vi "Test YOLO.vi"() -> ()   [LabVIEW 2017]
doc: "Created IvanLis by LabVIEW Portal\nProfile: http://labviewportal.org/memberlist.php?mode=viewprofile&u=987\neMail: IvanLisanov@gMail.com\nTelegram: https://t.me/IvanLis"
uses:
  libonnx_wrapper/libonnx_wrapper.lvlib
  process_YOLOv8/process_YOLOv8.lvlib
  libonnx_wrapper/TypeDef/IO.ctl
  libonnx_wrapper/TypeDef/Introspection.ctl
panel:
  out "Circles":cluster{"x":sgl, "y":sgl, "r":sgl}[](array[cluster])
  out "count":i32
  out "2D Picture":picture
  out "JPG file path":path=path "/home/ivan/LabVIEWData/ONNX/LabVIEW-ONNX_Runtime/image_for_test/1_1_2r_1_1_var10.jpg"
  out "Metadata":string[][](table)
  out "Introspection Output":T1
  out "Introspection Input":T1
  out "ONNX model path":path=path "/home/ivan/LabVIEWData/ONNX/LabVIEW-ONNX_Runtime/data/coins_detection.onnx"
  out "error out":errorcluster
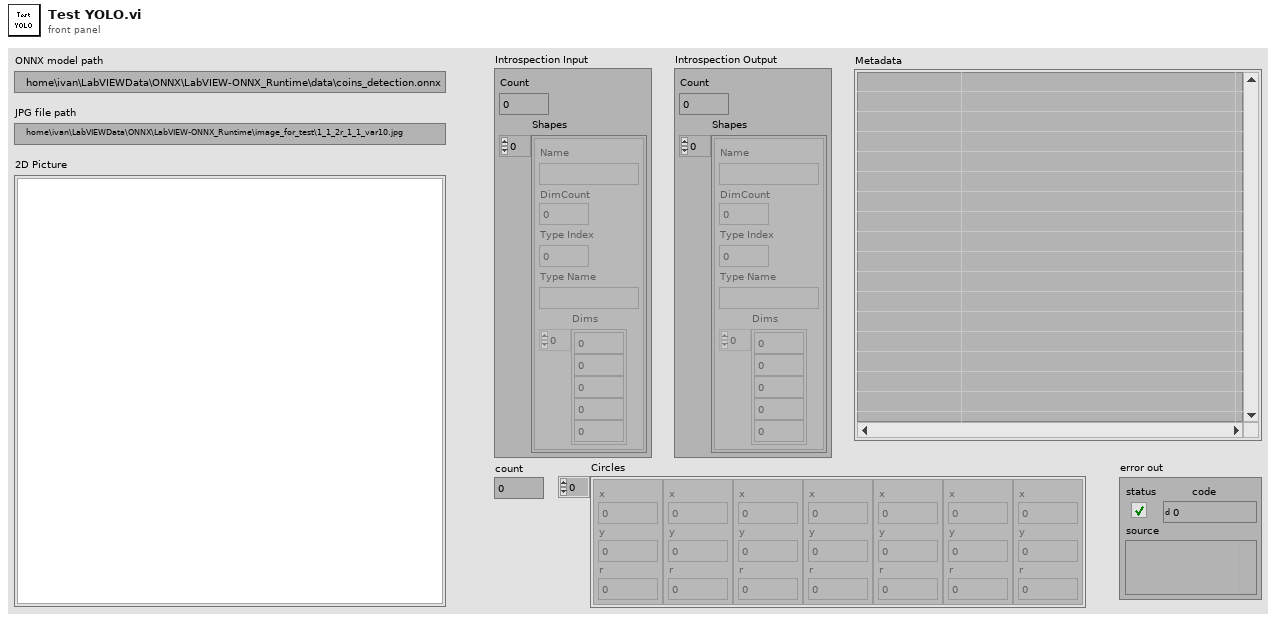
[diagram p1: front panel]
types:
  T1 = typedef "libonnx_wrapper.lvlib/Introspection.ctl" = cluster{"Count":i32, "Shapes":T2[]}
  T2 = typedef "libonnx_wrapper.lvlib/IO.ctl" = cluster{"Name":string, "DimCount":i32, "Type Index":i32, "Type Name":string, "Dims":i64[]}
  T3 = typedef "imagedata.ctl" = cluster{"image type":i32, "image depth":i32, "image":u8[], "mask":u8[], "colors":u32[], "Rectangle":cluster{"left":i16, "top":i16, "right":i16, "bottom":i16}}
  T4 = typedef "process_YOLOv8.lvlib/Circle.ctl" = cluster{"x":sgl, "y":sgl, "r":sgl}
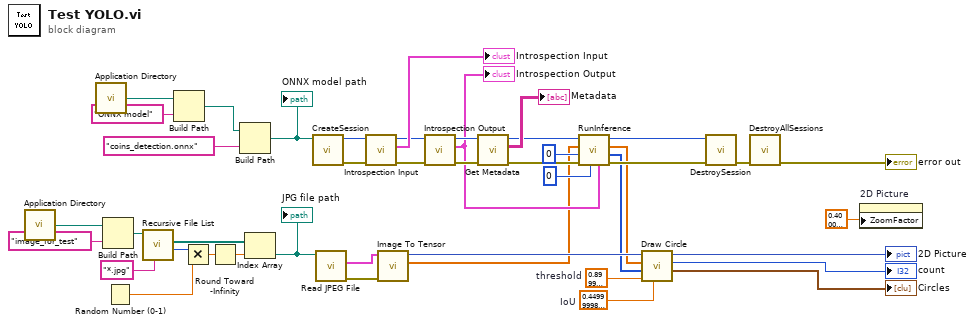
[diagram p0: block diagram]
diagram:
  w19 = sgl 0.45  # IoU
  w20 = sgl 0.9  # threshold
  n1 = call <vilib>:"Application Directory.vi"() -> ("Application Directory"=w9:path)
  n2 = call <vilib>:"Application Directory.vi"() -> ("Application Directory"=w14:path)
  n3 = Build Path(base path=w9, name or relative path="image_for_test") -> (appended path=w8:path)
  n4 = Random Number (0-1)() -> (number: 0 to 1=w6:dbl)
  n5 = call <vilib>:"Recursive File List.vi"("pattern"="*.jpg", "Folder Path"=w8) -> ("Number of Files"=w5:i32, "All Files in Dir"=w3:path[])  [unwired: 5 in, 3 out]
  n6 = Build Path(base path=w14, name or relative path="ONNX model") -> (appended path=w12:path)
  n7 = Multiply(x=w5, y=w6) -> (x*y=w4:dbl)
  n8 = Round Toward -Infinity(1:w4) -> (0:w2:dbl)
  n9 = Build Path(base path=w12, name or relative path="coins_detection.onnx") -> (appended path=w15:path)
  "ONNX model path" <- w15
  n10 = Index Array(array=w3, index=w2) -> (element=w1:path)
  "JPG file path" <- w1
  n11 = call "CreateSession.vi"("ONNX model path"=w15) -> ("error out"=w29:errorcluster, "session id out"=w30:i32)  [unwired: 9 in]
  n12 = call <vilib>:"Read JPEG File.vi"("path to JPEG file"=w1) -> ("error out"=w31:errorcluster, "image data"=w32:T3)  [unwired: 8 in, 1 out]
  n13 = call "Introspection Input.vi"("error in (no error)"=w29, "session id in"=w30) -> ("error out"=w41:errorcluster, "Introspection Input"=→"Introspection Input":T1, "session id out"=w42:i32)  [unwired: 7 in]
  n14 = call "Image To Tensor.vi"("error in (no error)"=w31, "image data"=w32) -> ("Data"=w11:sgl[], "image"=w26:picture)  [unwired: 7 in, 1 out]
  n15 = call "Introspection Output.vi"("error in (no error)"=w41, "session id in"=w42) -> ("error out"=w38:errorcluster, "Introspection Output"=w24:T1, "session id out"=w39:i32)  [unwired: 7 in]
  "Introspection Output" <- w24
  n16 = call "Get Metadata.vi"("error in (no error)"=w38, "session id in"=w39) -> ("error out"=w35:errorcluster, "Metadata"=→"Metadata":string[][], "session id out"=w36:i32)  [unwired: 7 in]
  n17 = call "RunInference.vi"("Introspection Output"=w24, "outputIndex"=0, "error in (no error)"=w35, "inputIndex"=0, "inputBuffer"=w11, "session id in"=w36) -> ("error out"=w28:errorcluster, "Dims"=w22:i64[], "outputBuffer"=w21:sgl[], "session id out"=w27:i32)  [unwired: 2 in]
  n18 = call "Draw Circle.vi"("IoU"=w19, "threshold"=w20, "dim"=w22, "data"=w21, "image in"=w26) -> ("Circles"=→"Circles":T4[], "count"=→"count":i32, "image out"=→"2D Picture":picture)  [unwired: 4 in]
  n19 = call "DestroySession.vi"("error in (no error)"=w28, "session id in"=w27) -> ("error out"=w44:errorcluster)  [unwired: 8 in, 1 out]
  n20 = call "DestroyAllSessions.vi"("error in (no error)"=w44) -> ("error out"=→"error out":errorcluster)  [unwired: 10 in]
  n21 = property on="2D Picture" class="Pict"("ZoomFactor"=sgl 0.4 ("Zoom Factor")) -> ()  [unwired: 2 in, 2 out]
